vi "Array2.vi"() -> ()   [LabVIEW 2020]
panel:
  out "min value":dbl
  out "max value":dbl
  in  "appended array 2":dbl[](array[numeric])
  out "output array":dbl[](array[numeric])
  in  "new element/subarray":dbl
  in  "index 2":i32
  out "subarray":dbl[](array[numeric])
  in  "length":i32
  in  "index":i32
  out "appended array":dbl[](array[numeric])
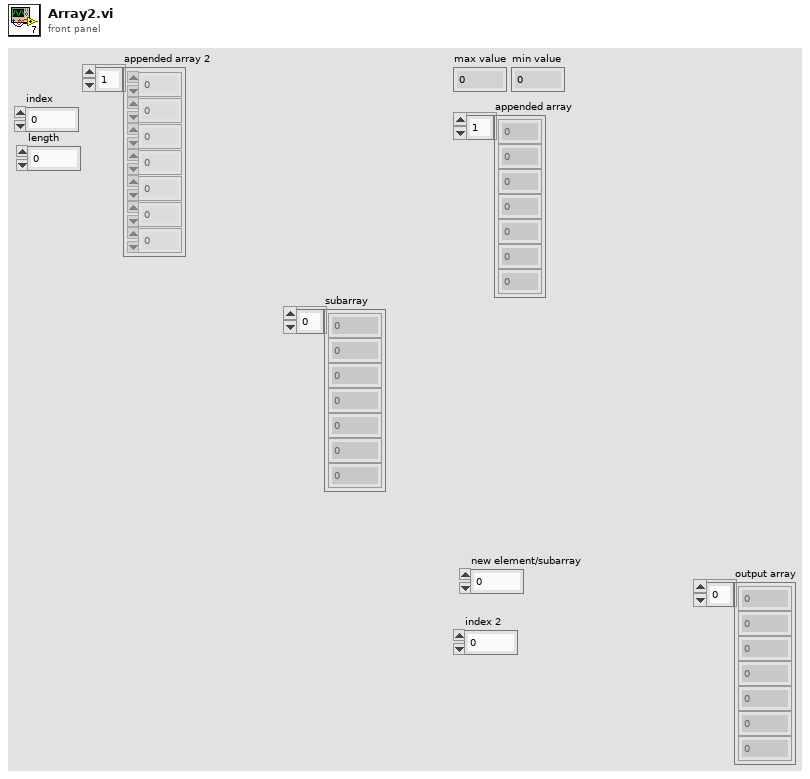
[diagram p1: front panel]
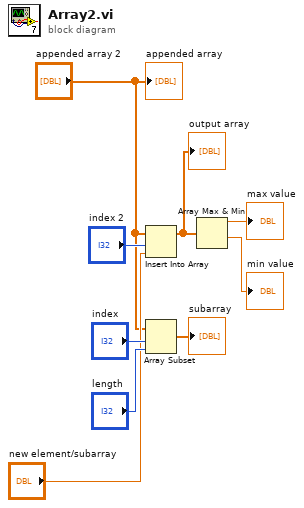
[diagram p0: block diagram]
diagram:
  n1 = Insert Into Array(array="appended array 2", index="index 2", new element="new element/subarray") -> (w3:dbl[])
  "output array" <- w3
  n2 = Array Subset(array="appended array 2", index="index", length="length") -> (→"subarray":dbl[])
  n3 = Array Max & Min(array=w3) -> (max value=→"max value":dbl, min value=→"min value":dbl)  [unwired: 2 out]
  "appended array" <- "appended array 2"
